vi "Fit.vi"(8 "error in (no error)":errorcluster caption="entrée d'erreur (pas d'erreur)", 9 "y":string[][](array[string]), 10 "X":string[][](array[string]), 11 "SkewedChi2Sampler.lvclass":refnum<class "SkewedChi2Sampler.lvclass">) -> (0 "error in (no error)":errorcluster caption="entrée d'erreur (pas d'erreur)", 2 "String Data":string, 3 "SkewedChi2Sampler.lvclass":refnum<class "SkewedChi2Sampler.lvclass">)   [LabVIEW 2020, in "SkewedChi2Sampler.lvclass"]
doc: "Fit the model with X.\n\nSamples random projection according to n_features.\n\n\nReturns : \n\n- String : OK"
uses:
  SkewedChi2Sampler.lvclass
  SkewedChi2Sampler.lvclass/SkewedChi2Sampler.ctl
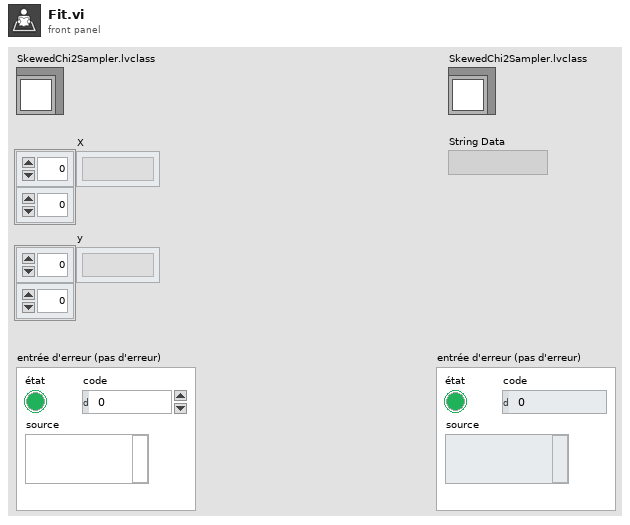
[diagram p1: front panel]
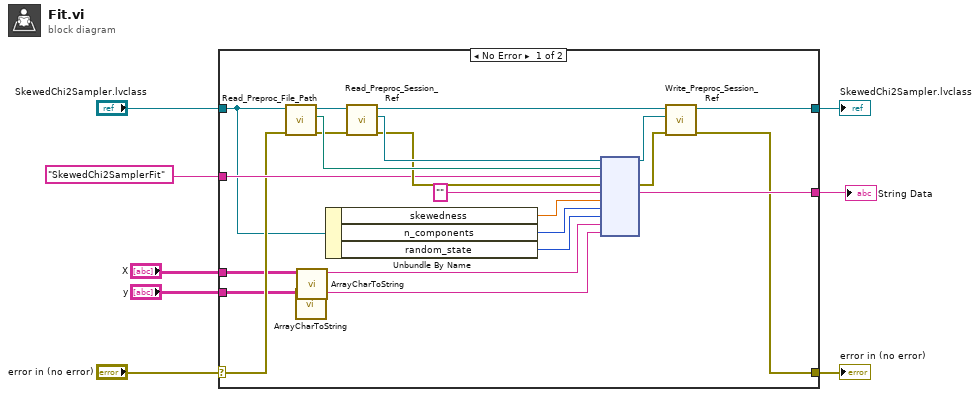
[diagram p0: block diagram]
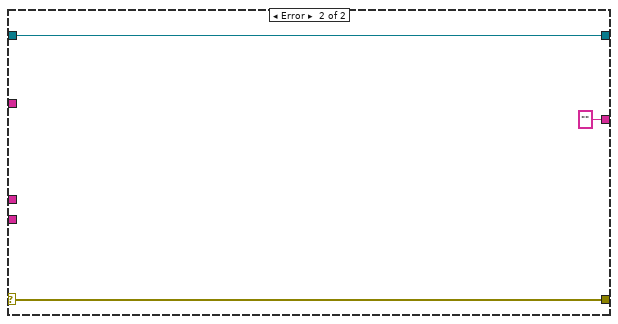
[diagram p2: hidden frame]
diagram:
  n1 = case shown="No Error" "error in (no error)" {
    selector: "error in (no error)" -> [w18 w33]
    tunnel: [w14 w33] -> w7
    tunnel: [w16 w32] -> w5
    tunnel: "SkewedChi2Sampler.lvclass" -> [w15 w32]
    tunnel: "SkewedChi2SamplerFit" ("Fonction") -> [w19 _]
    tunnel: "X" -> [w12 _]
    tunnel: [w17 ""] -> w2
    tunnel: "y" -> [w10 _]
    frame No Error {
      n2 = call-dynamic "Read_Preproc_File_Path.vi"("error in (no error)"=w18, "Python in"=w15) -> ("error out"=w25:errorcluster, "File_Path"=w28:path, "Python out"=w30:refnum<class "SkewedChi2Sampler.lvclass">)  [unwired: 7 in]
      n3 = call "ArrayCharToString.vi"("TAB"=w10) -> ("Instruction"=w9:string)  [unwired: 10 in]
      n4 = call "ArrayCharToString.vi"("TAB"=w12) -> ("Instruction"=w11:string)  [unwired: 10 in]
      n5 = Unbundle By Name(w15) -> ("skewedness"=w21:dbl, "n_components"=w20:i32, "random_state"=w13:i32)
      n6 = call-dynamic "Read_Preproc_Session_Ref.vi"("error in (no error)"=w25, "Python in"=w30) -> ("error out"=w26:errorcluster, "Session_ref"=w27:refnum<k35>, "Python out"=w29:refnum<class "SkewedChi2Sampler.lvclass">)  [unwired: 7 in]
      n7 = node(w27, w28, w19, w26, "", w21, w20, w13, w11, w9) -> (w22:refnum<k35>, w24:errorcluster, w17:string)  [unwired: 5 in, 2 out]
      n8 = call-dynamic "Write_Preproc_Session_Ref.vi"("error in (no error)"=w24, "Session_ref"=w22, "Python in"=w29) -> ("error out"=w14:errorcluster, "Python out"=w16:refnum<class "SkewedChi2Sampler.lvclass">)  [unwired: 7 in]
    }
    frame Error {
    }
  }
  "error in (no error)" <- w7
  "SkewedChi2Sampler.lvclass" <- w5
  "String Data" <- w2
